vi "host.conv.str.to.hex.vi"(11 "String":string="00, 0a, 35, 00, 01, 02, 60, a4, 4c, 63, f7, ea, 08, 00, 45, 00, 00, 5a, cb, 2a, 00, 00, 80, 11, eb, 11, c0, a8, 01, ca, c0, a8, 01, 3c, fb, 46, 17, 71, 00, 46, 19, 41, 54, 68, 69, 73, 20, 69, 73, 20, 74, 68, 65, 20, 6d, 65, 73, 73, 61, 67, 65, 2e, 20, 49, 74, 20, 77, 69, 6c, 6c, 20, 62, 65, 20, 72, 65, 70, 65, 61, 74, 65, 64, 2e, 20, 20, 54, 6f, 20, 47, 65, 6e, 65, 73, 79, 73, 20, 6f, 72, 20, 41, 72, 74, 79, 2e, 25, 7e, 94, 9c, ") -> (3 "Array 2":u8[](array[numeric])=[0, 10, 53, 0, 1, 2, 96, 164, 76, 99, 247, 234, 8, 0, 69, 0, 0, 90, 203, 42, 0, 0, 128, 17, 235, 17, 192, 168, 1, 202, 192, 168, 1, 60, 251, 70, 23, 113, 0, 70, 25, 65, 84, 104, 105, 115, 32, 105, 115, 32, 116, 104, 101, 32, 109, 101, 115, 115, 97, 103, 101, 46, 32, 73, 116, 32, 119, 105, 108, 108, 32, 98, 101, 32, 114, 101, 112, 101, 97, 116, 101, 100, 46, 32, 32, 84, 111, 32, 71, 101, 110, 101, 115, 121, 115, 32, 111, 114, 32, 65, 114, 116, 121, 46, 37, 126, 148, 156] format="%.0x")   [LabVIEW 2020]
panel:
  out "Array":string[](array[string])=["00", "0a", "35", "00", "01", "02", "60", "a4", "4c", "63", "f7", "ea", "08", "00", "45", "00", "00", "5a", "cb", "2a", "00", "00", "80", "11", "eb", "11", "c0", "a8", "01", "ca", "c0", "a8", "01", "3c", "fb", "46", "17", "71", "00", "46", "19", "41", "54", "68", "69", "73", "20", "69", "73", "20", "74", "68", "65", "20", "6d", "65", "73", "73", "61", "67", "65", "2e", "20", "49", "74", "20", "77", "69", "6c", "6c", "20", "62", "65", "20", "72", "65", "70", "65", "61", "74", "65", "64", "2e", "20", "20", "54", "6f", "20", "47", "65", "6e", "65", "73", "79", "73", "20", "6f", "72", "20", "41", "72", "74", "79", "2e", "25", "7e", "94", "9c"]
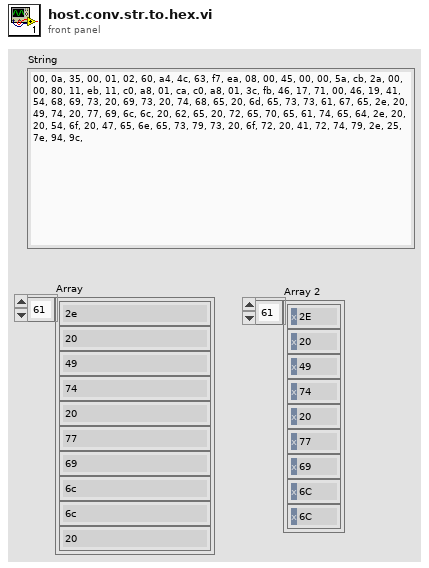
[diagram p1: front panel]
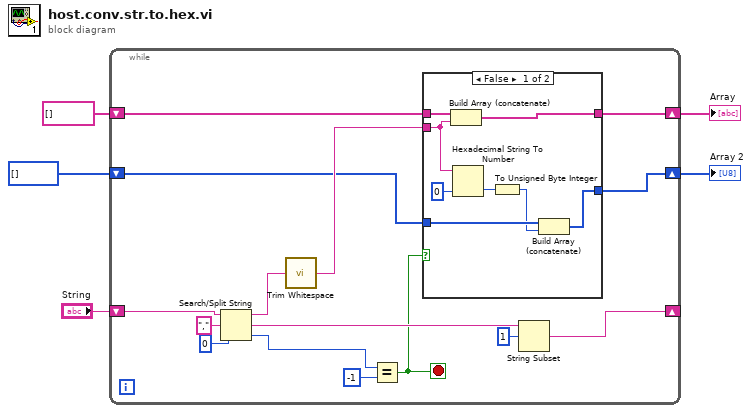
[diagram p0: block diagram]
diagram:
  n1 = while {
    shift-right: [w14] -> _
    shift-left: "String" -> [w19]
    shift-right: [w9] -> w3
    shift-left: string[] [] -> [w11]
    shift-right: [w7] -> w1
    shift-left: u8[] [] -> [w6]
    stop <- w8 stop-if-true
    n2 = Search/Split String(string=w19, search string/char (-)=",", offset (0)=0) -> (substring before match=w13:string, match + rest of string=w17:string, offset of match=w15:i32)
    n3 = call <vilib>:"Trim Whitespace.vi"("string"=w13) -> ("trimmed string"=w10:string)  [unwired: 1 in]
    n4 = Equal?(x=w15, y=-1) -> (x = y?=w8:bool)
    n5 = case shown="False" w8 {
      tunnel: w11 -> [w28 w30]
      tunnel: w10 -> [w26 _]
      tunnel: [w27 w30] -> w9
      tunnel: [w23 w29] -> w7
      tunnel: w6 -> [w25 w29]
      frame False {
        n6 = Build Array (concatenate)(w28, w26) -> (w27:string[])
        n7 = Hexadecimal String To Number(string=w26, default (0uL)=u32 0 ("default (0 U32)")) -> (number=w24:u32)  [unwired: 1 in, 1 out]
        n8 = To Unsigned Byte Integer(number=w24) -> (unsigned 8bit integer=w21:u8)
        n9 = Build Array (concatenate)(w25, w21) -> (w23:u8[])
      }
      frame True {
      }
    }
    n10 = String Subset(string=w17, offset (0)=1) -> (substring=w14:string)  [unwired: 1 in]
  }
  "Array" <- w3
  "Array 2" <- w1
